vi "Draft.vi"() -> ()   [LabVIEW 2018]
uses:
  <vilib>/Utility/miscctls.llb/LVRowAndColumnUnsignedTypeDef.ctl
panel:
  out "Boolean 5":bool
  out "Boolean 4":bool
  in  "Boolean 2":bool
  in  "Array 1":dbl[](array[numeric])
  out "Class Name":string
  out "Value":variant
  out "Objects on Page[]":refnum<vi>[](array[refnum])
  in  "Array Ctrl":dbl[](array[numeric])=[1.0, 2.0, 3.0, 4.0]
  in  "Tab Control":enum32{"Page 1", "Page 2"}(tab)
  in  "Array":dbl[](array[numeric])
  in  "Boolean 3":bool
  out "Waveform Chart":dbl(graph)
  in  "Array 2":dbl[](array[numeric])
  in  "String":string="qweqweq"
  in  "Index Values":T1
  in  "Table Control":string[][](table)
  out "Boolean":bool
  in  "stop":bool
  in  "Numeric":u8
  out "Slide":u8(slide) scale=0.0..100.0
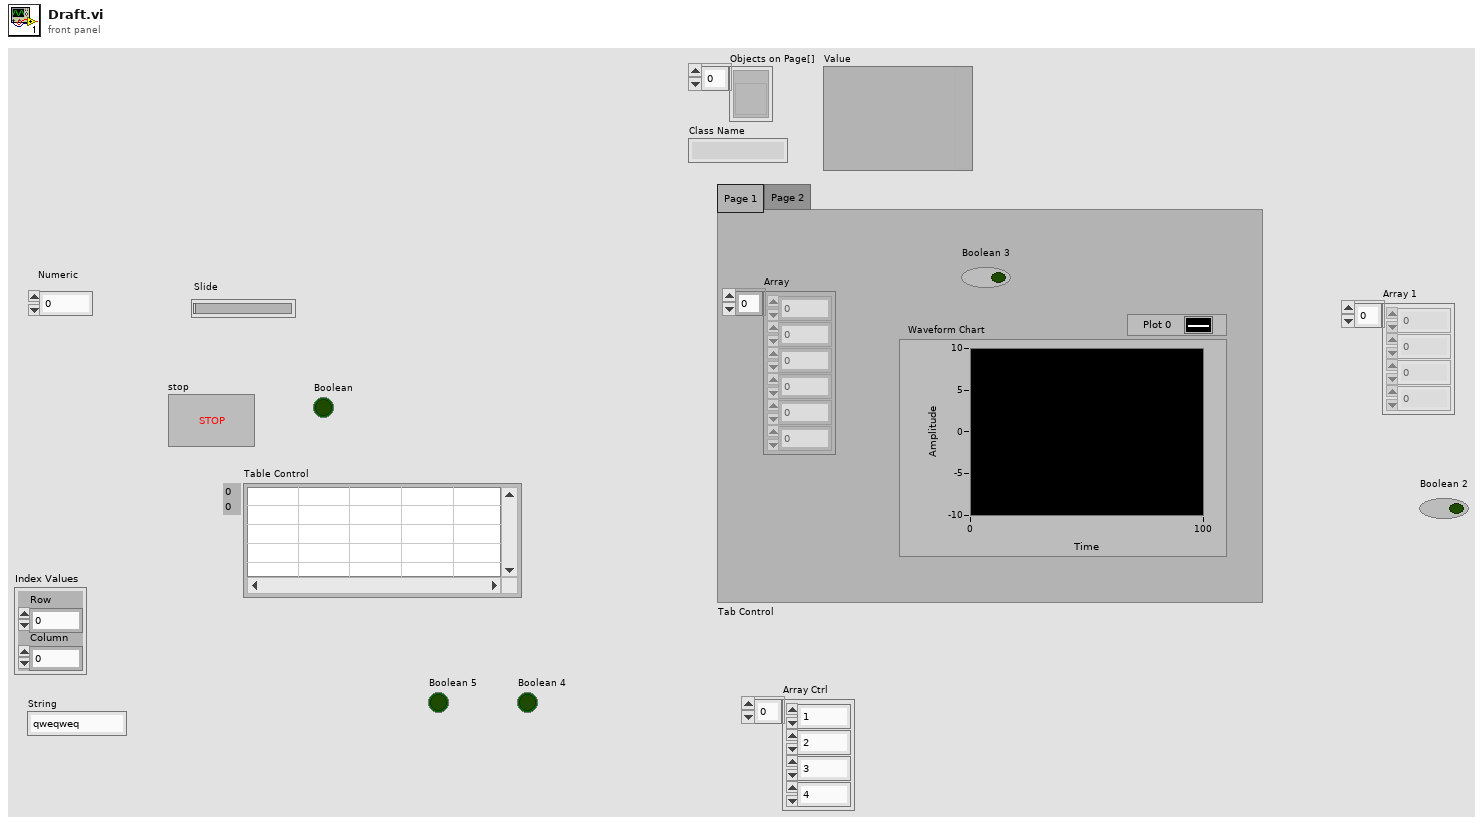
[diagram p1: front panel]
types:
  T1 = typedef "LVRowAndColumnUnsignedTypeDef.ctl" = cluster{"Row":u32, "Column":u32}
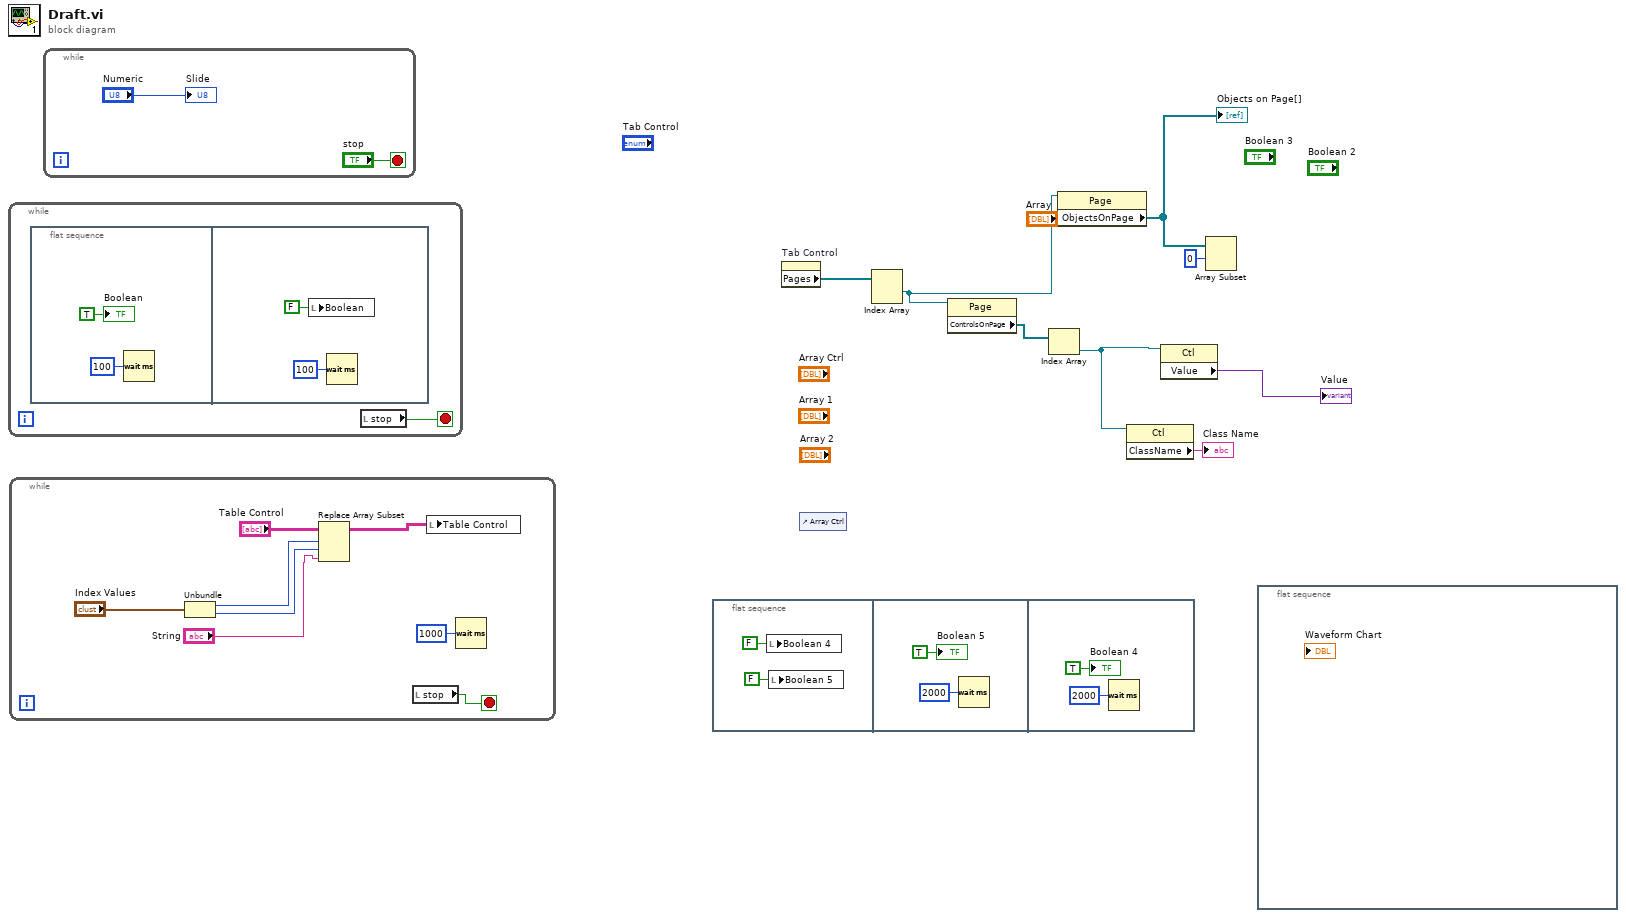
[diagram p0: block diagram]
diagram:
  n1 = while {
    stop <- w9 stop-if-true
    n2 = flat-sequence {
      frame #0 {
        n3 = Wait (ms)(milliseconds to wait=u32 100) -> ()  [unwired: 1 out]
        "Boolean" <- TRUE ("Boolean")
      }
      frame #1 {
        n4 = local write "Boolean"(FALSE ("Boolean")) -> ()
        n5 = Wait (ms)(milliseconds to wait=u32 100) -> ()  [unwired: 1 out]
      }
    }
    n6 = local read "stop"() -> (w9:bool)
  }
  n7 = while {
    stop <- w21 stop-if-true
    n8 = Unbundle("Index Values") -> ("Row"=w18:u32, "Column"=w17:u32)
    n9 = Replace Array Subset(array="Table Control", new element="String", index (row)=w18, index (col)=w17) -> (w16:string[][])
    n10 = local read "stop"() -> (w21:bool)
    n11 = local write "Table Control"(w16) -> ()
    n12 = Wait (ms)(milliseconds to wait=u32 1000) -> ()  [unwired: 1 out]
  }
  n13 = while {
    stop <- "stop" stop-if-true
    "Slide" <- "Numeric"
  }
  n14 = flat-sequence {
    frame #0 {
      n15 = local write "Boolean 4"(FALSE ("Boolean 4")) -> ()
      n16 = local write "Boolean 5"(FALSE ("Boolean 4")) -> ()
    }
    frame #1 {
      n17 = Wait (ms)(milliseconds to wait=u32 2000) -> ()  [unwired: 1 out]
      "Boolean 5" <- TRUE ("Boolean 4")
    }
    frame #2 {
      n18 = Wait (ms)(milliseconds to wait=u32 2000) -> ()  [unwired: 1 out]
      "Boolean 4" <- TRUE ("Boolean 4")
    }
  }
  n19 = property on="Tab Control" class="TabCtl (strict)"() -> ("Pages"=w8:refnum<vi>[])  [unwired: 2 in, 2 out]
  n20 = control-ref of="Array Ctrl"() -> ()  [unwired: 1 out]
  n21 = Index Array(array=w8) -> (element #1=w7:refnum<vi>)  [unwired: 2 in, 1 out]
  n22 = property class="Page"(reference=w7) -> ("ControlsOnPage"=w4:refnum<vi>[])  [unwired: 1 in, 2 out]
  n23 = Index Array(array=w4) -> (element=w2:refnum<vi>)  [unwired: 1 in]
  n24 = property class="Page"(reference=w7) -> ("ObjectsOnPage"=w6:refnum<vi>[])  [unwired: 1 in, 2 out]
  "Objects on Page[]" <- w6
  n25 = property class="Ctl"(reference=w2) -> ("ClassName"=→"Class Name":string)  [unwired: 1 in, 2 out]
  n26 = property class="Ctl"(reference=w2) -> ("Value"=→"Value":variant)  [unwired: 1 in, 2 out]
  n27 = Array Subset(array=w6, index=0) -> ()  [unwired: 1 in, 1 out]
  n28 = flat-sequence {
    frame #0 {
    }
  }
